vi "calculate current depth.vi"(11 "Cluster in":T1) -> (3 "Cluster out":T1)   [LabVIEW 2016]
uses:
  Waterloo DAQ/controls/Kpro hydraulic measurement cluster.ctl
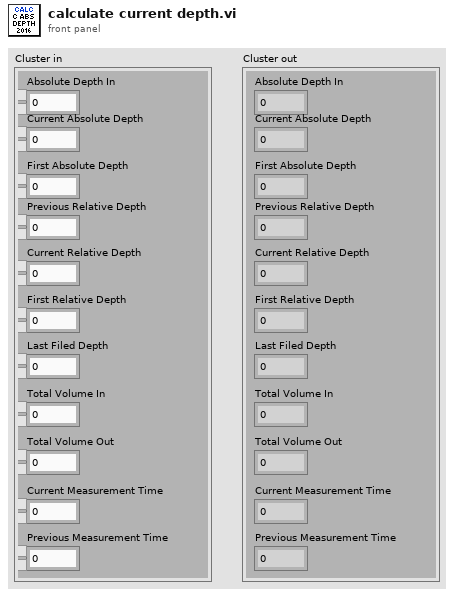
[diagram p1: front panel]
types:
  T1 = typedef "Kpro hydraulic measurement cluster.ctl" = cluster{"Absolute Depth In":dbl, "Current Absolute Depth":dbl, "First Absolute Depth":dbl, "Previous Relative Depth":dbl, "Current Relative Depth":dbl, "First Relative Depth":dbl, "Last Filed Depth":dbl, "Total Volume In":dbl, "Total Volume Out":dbl, "Current Measurement Time":dbl, "Previous Measurement Time":dbl}
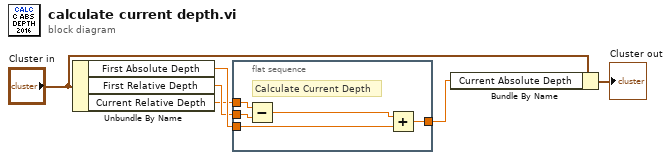
[diagram p0: block diagram]
diagram:
  n1 = Unbundle By Name("Cluster in") -> ("First Absolute Depth"=w3:dbl, "First Relative Depth"=w2:dbl, "Current Relative Depth"=w1:dbl)
  n2 = flat-sequence {
    tunnel: w2 -> [w11]
    tunnel: w3 -> [w9]
    tunnel: w1 -> [w8]
    tunnel: [w7] -> w4
    frame #0 {
      # "Calculate Current Depth"
      n3 = Subtract(x=w8, y=w11) -> (x-y=w10:dbl)
      n4 = Add(x=w10, y=w9) -> (x+y=w7:dbl)
    }
  }
  n5 = Bundle By Name(cluster="Cluster in", "Current Absolute Depth"=w4) -> (→"Cluster out":T1)
